vi "LevyLab Instrument.Write Configuration File.vi"(8 "error in (no error)":errorcluster, 11 "Example Instrument in":refnum<class "LevyLab Instrument.lvclass">) -> (0 "error out":errorcluster, 3 "Example Instrument out":refnum<class "LevyLab Instrument.lvclass">)   [LabVIEW 2016, in "LevyLab Instrument.lvclass"]
uses:
  LevyLab Instrument.lvclass
  C:/user/patrick/hg/levylab_inst/lvsrc/SMOs/Instrument/Instrument.lvclass
  SMOs/Instrument/Instrument.lvclass/Instrument.ctl
  LevyLab Instrument.lvclass/LevyLab Instrument.ctl
  SMOs/Configuration/Configuration.lvclass
  SMOs/Instrument/Instrument.lvclass
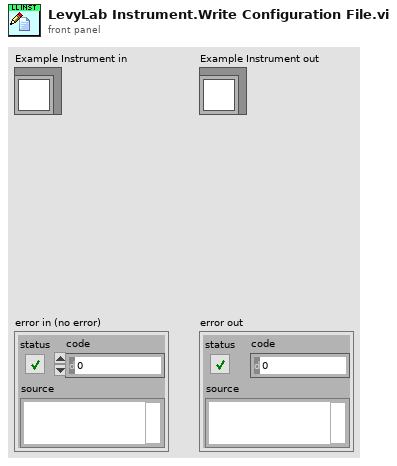
[diagram p1: front panel]
types:
  T1 = typedef "LevyLab Instrument.lvclass/LevyLab Instrument.Configuration--Cluster.ctl" = cluster{"Example Setting 1":dbl, "Example Setting 2":dbl, "Example Setting 3":string}
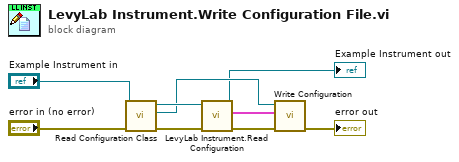
[diagram p0: block diagram]
diagram:
  n1 = call "Read Configuration Class.vi"("error in (no error)"="error in (no error)", "Instrument in"="Example Instrument in") -> ("error out"=w5:errorcluster, "Configuration.lvclass"=w8:refnum<class "Configuration.lvclass">, "Instrument out"=w9:refnum<class "LevyLab Instrument.lvclass">)  [unwired: 7 in]
  n2 = call "LevyLab Instrument.Read Configuration.vi"("error in (no error)"=w5, "Example Instrument in"=w9) -> ("error out"=w4:errorcluster, "Configuration"=w1:T1, "Example Instrument out"=→"Example Instrument out":refnum<class "LevyLab Instrument.lvclass">)  [unwired: 7 in]
  n3 = call "Write Configuration.vi"("error in (no error)"=w4, "Variant"=w1, "Configuration in"=w8) -> ("error out"=→"error out":errorcluster)  [unwired: 7 in, 1 out]
